vi "Vision Memory.vi"(8 "Distances in":T2(array[cluster])) -> (0 "Distances out":T2(array[cluster]))   [LabVIEW 2013]
uses:
  Program Files (x86)/National Instruments/LabVIEW 2013/examples/FRC/Vision/2014 Target Detection/TargetType.ctl
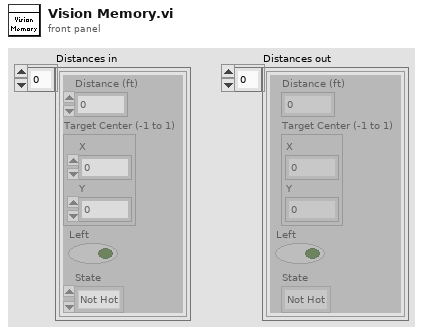
[diagram p1: front panel]
types:
  T1 = typedef "TargetType.ctl" = enum16{"Not Hot", "Hot"}
  T2 = cluster{"Distance (ft)":dbl, "Target Center (-1 to 1)":cluster{"X":dbl, "Y":dbl}, "Left":bool, "State":T1}[]
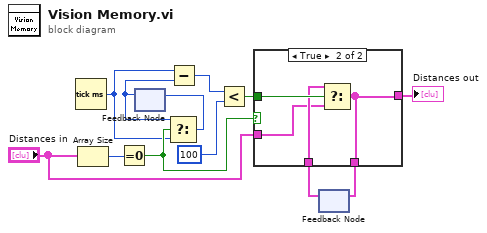
[diagram p0: block diagram]
diagram:
  n1 = Tick Count (ms)() -> (millisecond timer value=w3:u32)
  n2 = Array Size(array="Distances in") -> (size(s)=w5:i32)
  n3 = Equal To 0?(x=w5) -> (x = 0?=w8:bool)
  n4 = feedback #1() -> (w4:u32)  [unwired: 1 in]
  n5 = Select(t=w4, s=w8, f=w3) -> (s? t:f=w2:u32)
  n6 = feedback-in #1(w2) -> ()
  n7 = Subtract(x=w3, y=w4) -> (x-y=w6:u32)
  n8 = Less?(x=w6, y=u32 100) -> (x < y?=w9:bool)
  n9 = feedback #2() -> (w11:T2)  [unwired: 1 in]
  n10 = case shown="True" w8 {
    tunnel: "Distances in" -> [w13 w15]
    tunnel: w9 -> [_ w17]
    tunnel: [w13 w14] -> w10
    tunnel: w11 -> [_ w16]
    tunnel: [w13 w14] -> w12
    frame False {
    }
    frame True {
      n11 = Select(t=w16, s=w17, f=w15) -> (s? t:f=w14:T2)
    }
  }
  "Distances out" <- w12
  n12 = feedback-in #2(w10) -> ()
